vi "TMCM351-ReadLimit.vi"(3 "错误输入":errorcluster caption="错误输入（无错误）", 4 "通道":string(combo)="255", 5 "com in":refnum<visa-resource-name>) -> (0 "错误输出":errorcluster, 1 "Dout":i32, 2 "com out":refnum<visa-resource-name>)   [LabVIEW 2018]
panel:
  # "读取IO上的限位"
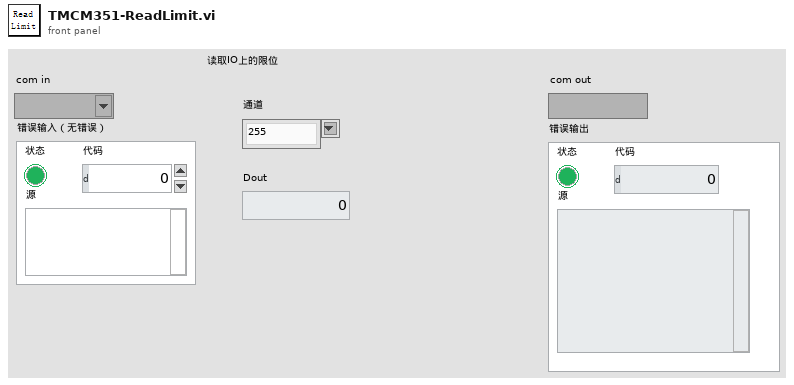
[diagram p1: front panel]
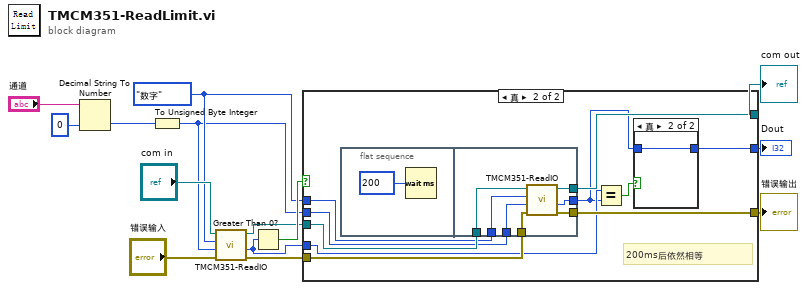
[diagram p0: block diagram]
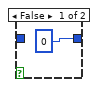
[diagram p3: hidden frame]
diagram:
  w6 = enum8{"数字", "模拟"}."数字" ("数据源")
  n1 = Decimal String To Number(string="通道", default (0L)=u8 0 ("默认(0 I32)")) -> (number=w10:u8)  [unwired: 1 in, 1 out]
  n2 = To Unsigned Byte Integer(number=w10) -> (unsigned 8bit integer=w5:u8)
  n3 = call "TMCM351-ReadIO.vi"("错误输入"="错误输入", "通道"=w5, "数据源"=w6, "com in"="com in") -> ("错误输出"=w7:errorcluster, "ReadOut"=w2:i32, "com out"=w8:refnum<visa-resource-name>)  [unwired: 1 in]
  n4 = Greater Than 0?(x=w2) -> (x > 0?=w9:bool)
  n5 = case shown="真" w9 {
    tunnel: w8 -> [w17 w27]
    tunnel: w7 -> [w16 w26]
    tunnel: w6 -> [_ w25]
    tunnel: w5 -> [_ w24]
    tunnel: [w16 w23] -> w4
    tunnel: [w17 w22] -> w3
    tunnel: w2 -> [w15 w21]
    tunnel: [w15 w18] -> w1
    frame False {
    }
    frame True {
      # "200ms后依然相等"
      n6 = flat-sequence {
        tunnel: w27 -> [w37]
        tunnel: w26 -> [w36]
        tunnel: w25 -> [w35]
        tunnel: w24 -> [w34]
        tunnel: [w33] -> w23
        tunnel: [w32] -> w22
        tunnel: [w31] -> w19
        frame #0 {
          n7 = Wait (ms)(milliseconds to wait=u32 200 ("等待时间（毫秒）")) -> ()  [unwired: 1 out]
        }
        frame #1 {
          n8 = call "TMCM351-ReadIO.vi"("错误输入"=w36, "通道"=w34, "数据源"=w35, "com in"=w37) -> ("错误输出"=w33:errorcluster, "ReadOut"=w31:i32, "com out"=w32:refnum<visa-resource-name>)  [unwired: 1 in]
        }
      }
      n9 = Equal?(x=w21, y=w19) -> (x = y?=w20:bool)
      n10 = case shown="真" w20 {
        tunnel: w19 -> [_ w29]
        tunnel: [0 w29] -> w18
        frame False {
        }
        frame True {
        }
      }
    }
  }
  "com out" <- w3
  "错误输出" <- w4
  "Dout" <- w1
